vi "McsaInitializeQbus.vi"(8 "error in (no error)":errorcluster) -> (0 "error out":errorcluster, 3 "Qbus out":refnum<class "Qbus.lvclass">)   [LabVIEW 2017]
uses:
  <vilib>/addons/Qbus/Qbus.lvclass
  <vilib>/addons/BlinkProcess/BlinkProcess.lvlib
  <vilib>/addons/TimerProcess/TimerProcess.lvlib
  <vilib>/addons/InsightCM/Devices/Shared/Common/ServerComm/ServerComm.lvlib
  <vilib>/addons/InsightCM/Devices/Shared/Common/Trigger/Trigger.lvlib
  <vilib>/addons/TraceLogger/TraceLogger.lvlib
  <vilib>/addons/InsightCM/Devices/Shared/Common/FileManager/FileManager.lvlib
  <vilib>/addons/InsightCM/Devices/Shared/Common/Controller/Controller.lvlib
  <vilib>/addons/InsightCM/Devices/Shared/Common/DataAccumulator/DataAccumulator.lvlib
  <vilib>/addons/InsightCM/Devices/Shared/Common/DeviceHealth/DeviceHealth.lvlib
  <vilib>/addons/InsightCM/Devices/Shared/Common/ModbusMaster/ModbusMaster.lvlib
  <vilib>/addons/InsightCM/Devices/Shared/Common/OpState/OpState.lvlib
  <vilib>/addons/InsightCM/Devices/Shared/Common/TrendAlarm/TrendAlarm.lvlib
  <vilib>/addons/InsightCM/Devices/Shared/Mcsa/McsaFpgaAcquisition/McsaFpgaAcquisition.lvlib
  <vilib>/addons/InsightCM/Devices/Shared/Mcsa/McsaVirtualChannel/McsaVirtualChannel.lvlib
  <vilib>/addons/InsightCM/Devices/Shared/Mcsa/McsaAnalysisLowUpdate/McsaAnalysisLowUpdate.lvlib
  <vilib>/addons/InsightCM/Devices/Shared/Mcsa/McsaAnalysisLowRate/McsaAnalysisLowRate.lvlib
  <vilib>/addons/InsightCM/Devices/Shared/Mcsa/McsaAnalysisHighRate/McsaAnalysisHighRate.lvlib
  <vilib>/addons/InsightCM/Devices/Shared/Mcsa/McsaStartupAnalysis/McsaStartupAnalysis.lvlib
  <vilib>/addons/InsightCM/Devices/Shared/Mcsa/McsaDataEventCreator/McsaDataEventCreator.lvlib
  <vilib>/addons/InsightCM/Devices/Shared/Mcsa/McsaFpgaBitfileManager/McsaFpgaBitfileManager.lvlib
  <vilib>/addons/InsightCM/Devices/Shared/Mcsa/McsaTestPanel/McsaTestPanel.lvlib
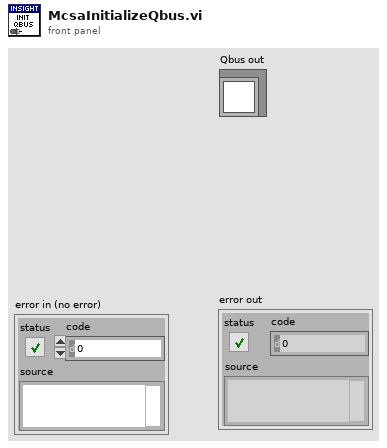
[diagram p1: front panel]
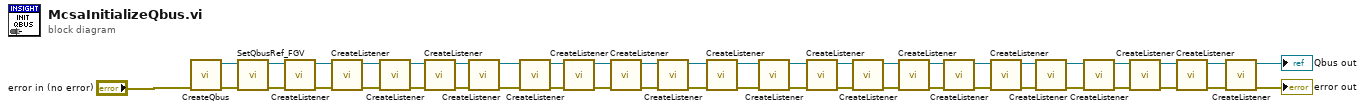
[diagram p0: block diagram]
diagram:
  n1 = call <vilib>:"CreateQbus.vi"("error in (no error)"="error in (no error)") -> ("error out"=w40:errorcluster, "Qbus"=w39:refnum<class "Qbus.lvclass">)  [unwired: 9 in]
  n2 = call <vilib>:"SetQbusRef_FGV.vi"("error in (no error)"=w40, "Qbus in"=w39) -> ("error out"=w38:errorcluster, "Qbus out"=w37:refnum<class "Qbus.lvclass">)  [unwired: 8 in]
  n3 = call <vilib>:"CreateListener.vi"("error in (no error)"=w38, "Qbus in"=w37) -> ("error out"=w42:errorcluster, "Qbus out"=w41:refnum<class "Qbus.lvclass">)  [unwired: 8 in]
  n4 = call <vilib>:"CreateListener.vi"("error in (no error)"=w42, "Qbus in"=w41) -> ("error out"=w31:errorcluster, "Qbus out"=w32:refnum<class "Qbus.lvclass">)  [unwired: 8 in]
  n5 = call <vilib>:"CreateListener.vi"("error in (no error)"=w31, "Qbus in"=w32) -> ("error out"=w30:errorcluster, "Qbus out"=w29:refnum<class "Qbus.lvclass">)  [unwired: 8 in]
  n6 = call <vilib>:"CreateListener.vi"("error in (no error)"=w30, "Qbus in"=w29) -> ("error out"=w14:errorcluster, "Qbus out"=w13:refnum<class "Qbus.lvclass">)  [unwired: 8 in]
  n7 = call <vilib>:"CreateListener.vi"("error in (no error)"=w14, "Qbus in"=w13) -> ("error out"=w27:errorcluster, "Qbus out"=w28:refnum<class "Qbus.lvclass">)  [unwired: 8 in]
  n8 = call <vilib>:"CreateListener.vi"("error in (no error)"=w27, "Qbus in"=w28) -> ("error out"=w26:errorcluster, "Qbus out"=w25:refnum<class "Qbus.lvclass">)  [unwired: 8 in]
  n9 = call <vilib>:"CreateListener.vi"("error in (no error)"=w26, "qbus in"=w25) -> ("error out"=w44:errorcluster, "qbus out"=w43:refnum<class "Qbus.lvclass">)  [unwired: 8 in]
  n10 = call <vilib>:"CreateListener.vi"("error in (no error)"=w44, "qbus"=w43) -> ("error out"=w5:errorcluster, "qbus out"=w6:refnum<class "Qbus.lvclass">)  [unwired: 8 in]
  n11 = call <vilib>:"CreateListener.vi"("error in (no error)"=w5, "Qbus"=w6) -> ("error out"=w8:errorcluster, "Qbus out"=w7:refnum<class "Qbus.lvclass">)  [unwired: 8 in]
  n12 = call <vilib>:"CreateListener.vi"("error in (no error)"=w8, "Qbus"=w7) -> ("error out"=w9:errorcluster, "Qbus out"=w10:refnum<class "Qbus.lvclass">)  [unwired: 8 in]
  n13 = call <vilib>:"CreateListener.vi"("error in (no error)"=w9, "Qbus"=w10) -> ("error out"=w12:errorcluster, "Qbus out"=w11:refnum<class "Qbus.lvclass">)  [unwired: 8 in]
  n14 = call <vilib>:"CreateListener.vi"("error in (no error)"=w12, "Qbus in"=w11) -> ("error out"=w20:errorcluster, "Qbus out"=w19:refnum<class "Qbus.lvclass">)  [unwired: 8 in]
  n15 = call <vilib>:"CreateListener.vi"("error in (no error)"=w20, "Qbus in"=w19) -> ("error out"=w24:errorcluster, "Qbus out"=w21:refnum<class "Qbus.lvclass">)  [unwired: 8 in]
  n16 = call <vilib>:"CreateListener.vi"("error in (no error)"=w24, "Qbus in"=w21) -> ("error out"=w23:errorcluster, "Qbus out"=w22:refnum<class "Qbus.lvclass">)  [unwired: 8 in]
  n17 = call <vilib>:"CreateListener.vi"("error in (no error)"=w23, "Qbus in"=w22) -> ("error out"=w36:errorcluster, "Qbus out"=w35:refnum<class "Qbus.lvclass">)  [unwired: 8 in]
  n18 = call <vilib>:"CreateListener.vi"("error in (no error)"=w36, "Qbus"=w35) -> ("error out"=w16:errorcluster, "Qbus out"=w15:refnum<class "Qbus.lvclass">)  [unwired: 8 in]
  n19 = call <vilib>:"CreateListener.vi"("error in (no error)"=w16, "Qbus in"=w15) -> ("error out"=w17:errorcluster, "Qbus out"=w18:refnum<class "Qbus.lvclass">)  [unwired: 8 in]
  n20 = call <vilib>:"CreateListener.vi"("error in (no error)"=w17, "Qbus in"=w18) -> ("error out"=w33:errorcluster, "Qbus out"=w34:refnum<class "Qbus.lvclass">)  [unwired: 8 in]
  n21 = call <vilib>:"CreateListener.vi"("error in (no error)"=w33, "Qbus in"=w34) -> ("error out"=w46:errorcluster, "Qbus out"=w47:refnum<class "Qbus.lvclass">)  [unwired: 8 in]
  n22 = call <vilib>:"CreateListener.vi"("error in (no error)"=w46, "qbus in"=w47) -> ("error out"=w4:errorcluster, "qbus out"=w3:refnum<class "Qbus.lvclass">)  [unwired: 8 in]
  n23 = call <vilib>:"CreateListener.vi"("error in (no error)"=w4, "Qbus"=w3) -> ("error out"=→"error out":errorcluster, "Qbus out"=→"Qbus out":refnum<class "Qbus.lvclass">)  [unwired: 8 in]
